vi "Config Filter.vi"(8 "error in (no error)":errorcluster, 9 "low cutoff freq: fl":dbl=10.0 format="%0.3f", 10 "sampling freq: fs":dbl=1000.0 format="%0.2f", 11 "Sig_AI in":refnum<class "AI.lvclass">) -> (0 "error out":errorcluster, 3 "Sig_AI out":refnum<class "AI.lvclass">)   [LabVIEW 2019, in "AI.lvclass"]
uses:
  AI.lvclass
  AI.lvclass/AI.ctl
  <vilib>/Analysis/NI_AALBase.lvlib
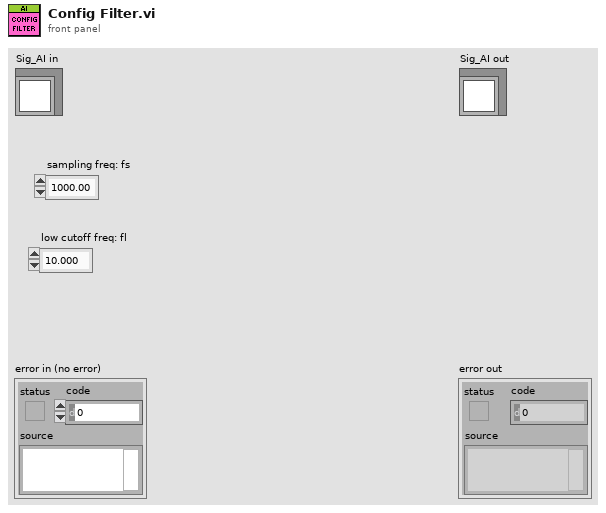
[diagram p1: front panel]
types:
  T1 = cluster{"filter structure":enum32{"IIR 2nd Order", "IIR 4th Order"}, "Reverse Coefficients":dbl[], "Forward Coefficients":dbl[]}
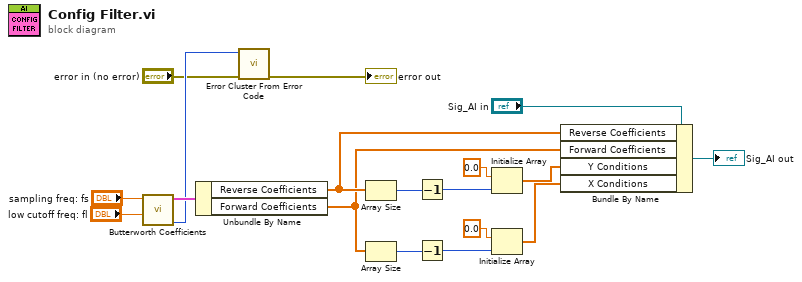
[diagram p0: block diagram]
diagram:
  n1 = call <vilib>:"Butterworth Coefficients.vi"("low cutoff freq: fl"="low cutoff freq: fl", "sampling freq: fs"="sampling freq: fs") -> ("error"=w14:i32, "IIR Filter Cluster"=w16:T1)  [unwired: 8 in]
  n2 = Unbundle By Name(w16) -> ("Reverse Coefficients"=w10:dbl[], "Forward Coefficients"=w9:dbl[])
  n3 = call <vilib>:"Error Cluster From Error Code.vi"("error in (no error)"="error in (no error)", "error code (0)"=w14) -> ("error out"=→"error out":errorcluster)  [unwired: 7 in]
  n4 = Array Size(array=w10) -> (size(s)=w8:i32)
  n5 = Array Size(array=w9) -> (size(s)=w7:i32)
  n6 = Decrement(x=w8) -> (x-1=w3:i32)
  n7 = Decrement(x=w7) -> (x-1=w6:i32)
  n8 = Initialize Array(0.0 ("element"), w3) -> (w1:dbl[])
  n9 = Initialize Array(0.0 ("element"), w6) -> (w2:dbl[])
  n10 = Bundle By Name(cluster="Sig_AI in", "Reverse Coefficients"=w10, "Forward Coefficients"=w9, "Y Conditions"=w1, "X Conditions"=w2) -> (→"Sig_AI out":refnum<class "AI.lvclass">)
